vi "Command_Auto_Intaking.vi"(7 "Startup":bool, 8 "timeout":dbl=20.0, 9 "target heading":dbl, 10 "speed":dbl=15.0) -> (1 "Turn Speed(rad/s)":dbl=0.021240234375, 2 "Linear Speed(in/s)":dbl=15.0, 4 "Reint":bool, 6 "Completed":bool)   [LabVIEW 2019]
uses:
  Auto Utilities/Command_Execution_State.ctl
  Subsystems/Sensing/Sensor_Values.vi
panel:
  in  "acceptable_line_error":dbl=1.0
  in  "deflection_delay(ms)":u32=200
  out "balls_grabbed":i8=11
  in  "deflection_angle":dbl=30.0
  out "Balls Grabbed":i8=11
  in  "Turn Kd":dbl
  in  "Turn Kp":dbl=0.05
  in  "Max PID output":dbl=5.0
  out "Waveform Chart":cluster{"Goal Wheel Position":dbl, dbl}(graph)
  in  "Cam Kd":dbl
  in  "Cam Kp":dbl=0.05
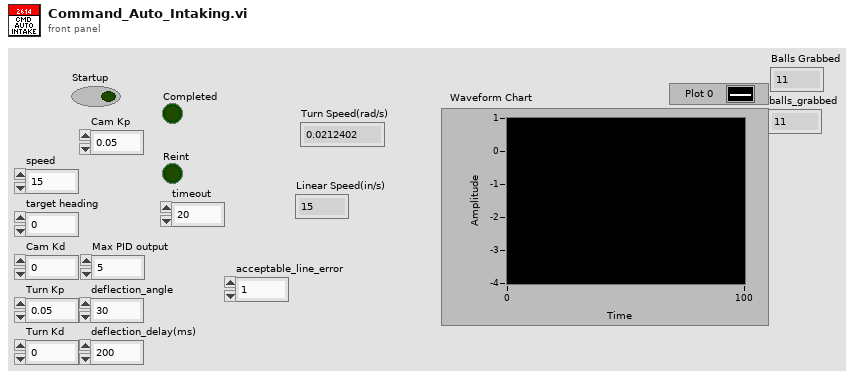
[diagram p1: front panel]
types:
  T1 = typedef "Command_Execution_State.ctl" = enum16{"Initialize", "Execute", "Finish"}
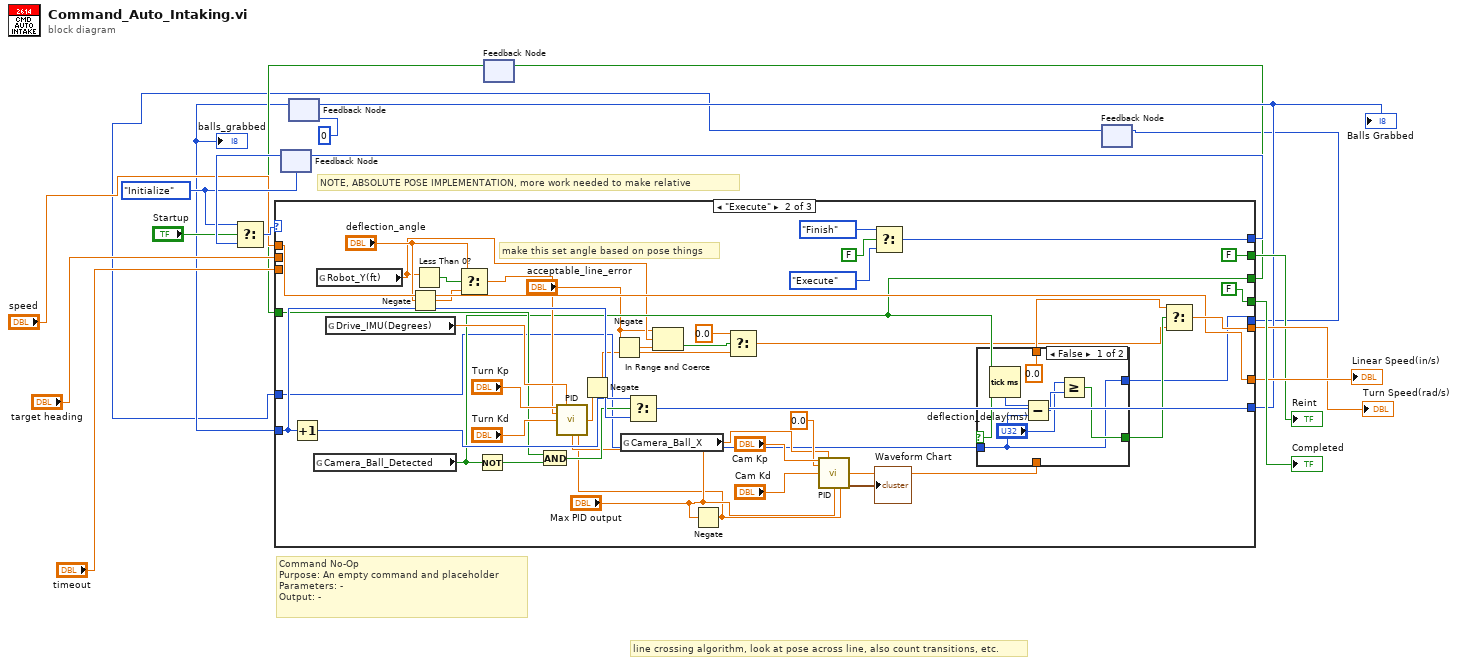
[diagram p0: block diagram]
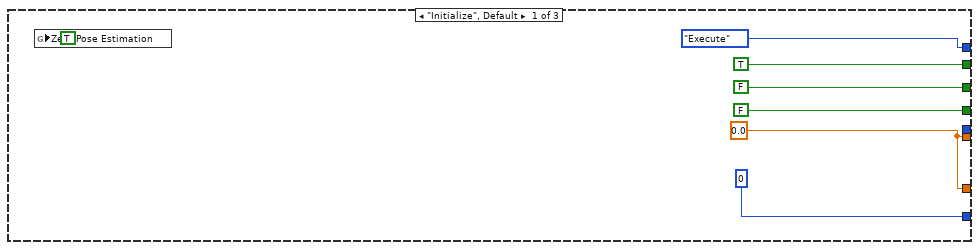
[diagram p2: hidden frame]
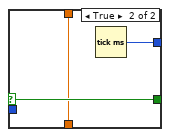
[diagram p3: hidden frame]
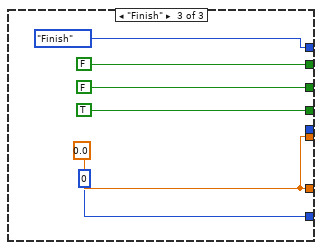
[diagram p4: hidden frame]
diagram:
  w14 = Command_Execution_State."Initialize" ("Play State")
  # "line crossing algorithm, look at pose across line, also count transitions, etc."
  # "NOTE, ABSOLUTE POSE IMPLEMENTATION, more work needed to make relative"
  # "Command No-Op\nPurpose: An empty command and placeholder\nParameters: -\nOutput: -"
  n1 = feedback #1(w14) -> (w17:T1)
  n2 = Select(t=w14, s="Startup", f=w17) -> (s? t:f=w19:T1)
  n3 = feedback #2(i8 0 ("8bit integer")) -> (w3:i8)
  "balls_grabbed" <- w3
  n4 = feedback #3() -> (w4:bool)  [unwired: 1 in]
  n5 = feedback #4() -> (w1:u32)  [unwired: 1 in]
  n6 = case shown="\"Execute\"" w19 {
    tunnel: [Command_Execution_State."Execute" ("Play State") w66 Command_Execution_State."Finish" ("Play State")] -> w18
    tunnel: [FALSE FALSE TRUE] -> w16
    tunnel: [TRUE FALSE FALSE] -> w8
    tunnel: "speed" -> [_ w44 _]
    tunnel: "target heading" -> [_ _ _]
    tunnel: "timeout" -> [_ _ _]
    tunnel: [w23 w44 w80] -> w10
    tunnel: [w23 w57 w80] -> w9
    tunnel: w3 -> [_ w51 _]
    tunnel: [i8 0 ("8bit integer") w52 i8 0 ("8bit integer")] -> w6
    tunnel: [FALSE ("Camera_Ball_Detected") w39 FALSE ("Camera_Ball_Detected")] -> w5
    tunnel: w4 -> [_ w48 _]
    tunnel: [_ w37 _] -> w2
    tunnel: w1 -> [_ w36 _]
    frame "Initialize", Default {
      w23 = 0.0 ("Linear Speed(in/s)")
      n7 = global write "Sensor_Values.vi" "Zero Pose Estimation"(TRUE ("Zero Pose Estimation")) -> ()
    }
    frame "Execute" {
      # "make this set angle based on pose things"
      n8 = Increment(x=w51) -> (x+1=w50:i8)
      n9 = global read "Sensor_Values.vi" "Camera_Ball_Detected"() -> (w39:bool)
      n10 = global read "Sensor_Values.vi" "Robot_Y(ft)"() -> (w30:dbl)
      n11 = global read "Sensor_Values.vi" "Drive_IMU(Degrees)"() -> (w56:dbl)
      n12 = Negate(x="deflection_angle") -> (-x=w40:dbl)
      n13 = Less Than 0?(x=w30) -> (x < 0?=w42:bool)
      n14 = Select(t="deflection_angle", s=w42, f=w40) -> (s? t:f=w43:dbl)
      n15 = Not(x=w39) -> (.not. x?=w47:bool)
      n16 = And(x=w48, y=w47) -> (x .and. y?=w49:bool)
      n17 = Negate(x="acceptable_line_error") -> (-x=w27:dbl)
      n18 = global read "Sensor_Values.vi" "Camera_Ball_X"() -> (w60:dbl)
      n19 = Select(t=w50, s=w49, f=w51) -> (s? t:f=w52:i8)
      n20 = In Range and Coerce(upper limit="acceptable_line_error", x=w30, lower limit=w27) -> (In Range?=w31:bool)  [unwired: 1 out]
      n21 = Negate(x="Max PID output") -> (-x=w45:dbl)
      n22 = call "PID.vi"("Kp"="Turn Kp", "Process Variable"=w56, "Goal"=w43, "Kd"="Turn Kd", "Max Ouput"="Max PID output", "Min Output"=w45) -> ("Command"=w55:dbl)  [unwired: 7 in, 2 out]
      n23 = Negate(x=w55) -> (-x=w33:dbl)
      n24 = Select(t=0.0, s=w31, f=w33) -> (s? t:f=w32:dbl)
      n25 = call "PID.vi"("Kp"="Cam Kp", "Process Variable"=w60, "Goal"=0.0, "Kd"="Cam Kd", "Max Ouput"="Max PID output", "Min Output"=w45) -> ("Command"=w35:dbl, "PID Tracking"=→"Waveform Chart":cluster{"Goal Wheel Position":dbl, dbl})  [unwired: 7 in, 1 out]
      n26 = Select(t=Command_Execution_State."Finish" ("Play State"), s=FALSE, f=Command_Execution_State."Execute" ("Play State")) -> (s? t:f=w66:T1)
      n27 = case shown="False" w39 {
        selector: w39 -> [_ w77]
        tunnel: [w74 w77] -> w38
        tunnel: [w72 w76] -> w37
        tunnel: w36 -> [w72 _]
        tunnel: w35 -> [_ w75]
        tunnel: [0.0 ("Command") w75] -> w34
        frame False {
          n28 = Tick Count (ms)() -> (millisecond timer value=w73:u32)
          n29 = Subtract(x=w73, y=w72) -> (x-y=w71:u32)
          n30 = Greater Or Equal?(x="deflection_delay(ms)", y=w71) -> (x >= y?=w74:bool)
        }
        frame True {
          n31 = Tick Count (ms)() -> (millisecond timer value=w76:u32)
        }
      }
      n32 = Select(t=w34, s=w38, f=w32) -> (s? t:f=w57:dbl)
    }
    frame "Finish" {
      w80 = 0.0 ("Linear Speed(in/s)")
    }
  }
  "Completed" <- w16
  "Reint" <- w8
  "Linear Speed(in/s)" <- w10
  "Turn Speed(rad/s)" <- w9
  "Balls Grabbed" <- w6
  n33 = feedback-in #1(w18) -> ()
  n34 = feedback-in #2(w6) -> ()
  n35 = feedback-in #3(w5) -> ()
  n36 = feedback-in #4(w2) -> ()
